vi "Init Control.vi"(5 "Group":refnum<class "Group DBL.lvclass">, 6 "Period ms":i64, 7 "VolatusAPI":refnum<class "VolatusAPI.lvclass">, 8 "error in (no error)":errorcluster, 9 "Control MsgQ":refnum<class "MessageQ.lvclass">, 10 "Config Element":refnum<class "Config Element.lvclass">, 11 "Valve in":refnum<class "BangBangControl.lvclass">) -> (0 "error out":errorcluster, 3 "Valve out":refnum<class "BangBangControl.lvclass">)   [LabVIEW 2020, in "VolatusControl.lvlib" / "BangBangControl.lvclass"]
uses:
  BangBangControl.lvclass
  lv-cdm/CDM-Config/Config Element/Config Element.lvclass
  Volatus/VolatusAPI/VolatusAPI.lvclass
  Volatus/MessageQ/MessageQ.lvclass
  lv-vecto/Vecto/Group DBL/Group DBL.lvclass
  C:/dev/lv20CE/relink/lv-vecto/Vecto/Group/Group.lvclass
  PV Calc.ctl
  BangBangControl.lvclass/BangBangControl.ctl
  VolatusControl.lvlib
  lv-vecto/Vecto/Group/Group.lvclass
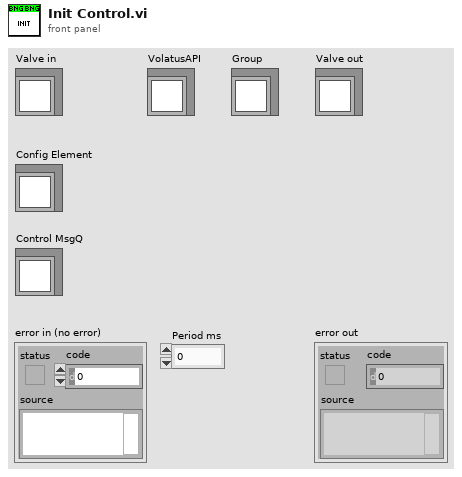
[diagram p1: front panel]
types:
  T1 = typedef "VolatusControl.lvlib/BangBangControl.lvclass/PV Calc.ctl" = enum16{"Average", "Median", "Max", "Min"}
  T2 = typedef "CDM-Config.lvlib/Value Type.ctl" = enum16{"String", "Number", "Bool", "Object", "Array"}
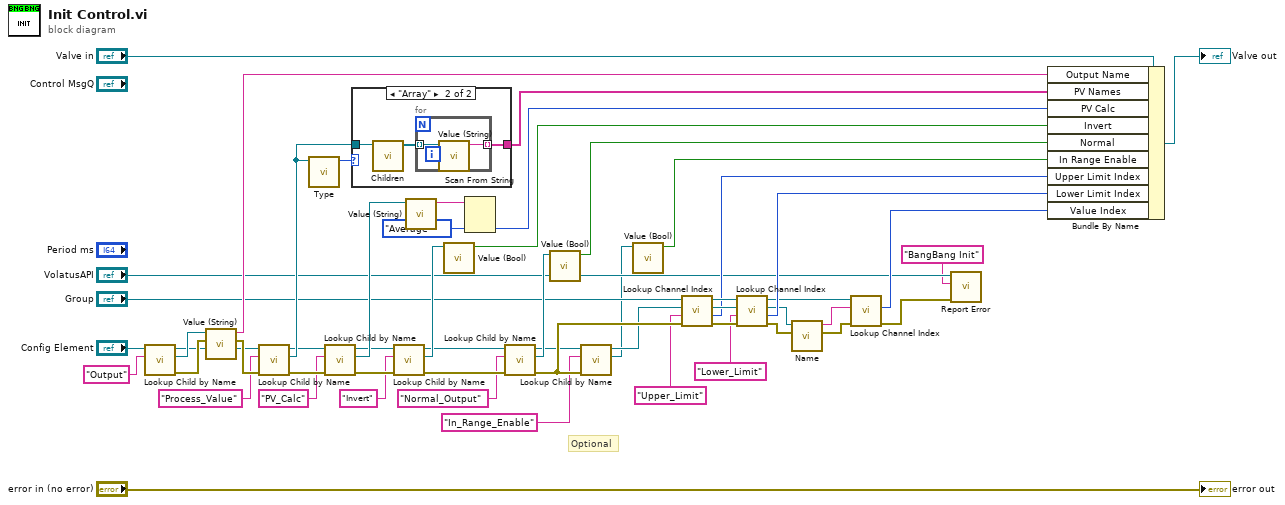
[diagram p0: block diagram]
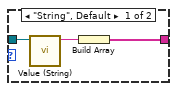
[diagram p2: hidden frame]
diagram:
  # "Optional"
  n1 = call "Lookup Child by Name.vi"("Name"="Output", "Config Element in"="Config Element") -> ("error out"=w44:errorcluster, "Child"=w45:refnum<class "Config Element.lvclass">, "Config Element out"=w41:refnum<class "Config Element.lvclass">)  [unwired: 6 in, 1 out]
  n2 = call "Value (String).vi"("error in (no error)"=w44, "Config Element in"=w45) -> ("error out"=w50:errorcluster, "String Value"=w42:string)  [unwired: 8 in]
  n3 = call "Lookup Child by Name.vi"("error in (no error)"=w50, "Name"="Process_Value", "Config Element in"=w41) -> ("error out"=w51:errorcluster, "Child"=w38:refnum<class "Config Element.lvclass">, "Config Element out"=w33:refnum<class "Config Element.lvclass">)  [unwired: 5 in, 1 out]
  n4 = call "Type.vi"("Config Element in"=w38) -> ("Value Type"=w39:T2)  [unwired: 9 in, 1 out]
  n5 = call "Lookup Child by Name.vi"("error in (no error)"=w51, "Name"="PV_Calc", "Config Element in"=w33) -> ("error out"=w52:errorcluster, "Child"=w32:refnum<class "Config Element.lvclass">, "Config Element out"=w29:refnum<class "Config Element.lvclass">)  [unwired: 5 in, 1 out]
  n6 = case shown="\"Array\"" w39 {
    tunnel: w38 -> [w57 w60]
    tunnel: [w55 w58] -> w37
    frame "String", Default {
      n7 = call "Value (String).vi"("Config Element in"=w57) -> ("String Value"=w56:string)  [unwired: 9 in, 1 out]
      n8 = Build Array(w56) -> (w55:string[])
    }
    frame "Array" {
      n9 = call "Children.vi"("Config Element in"=w60) -> ("Elements"=w59:refnum<class "Config Element.lvclass">[])  [unwired: 9 in, 1 out]
      n10 = for {
        tunnel: w59 -> [w62] mode=indexing
        tunnel: [w61] -> w58 mode=indexing
        n11 = call "Value (String).vi"("Config Element in"=w62) -> ("String Value"=w61:string)  [unwired: 9 in, 1 out]
      }
    }
  }
  n12 = call "Lookup Child by Name.vi"("error in (no error)"=w52, "Name"="Invert", "Config Element in"=w29) -> ("error out"=w53:errorcluster, "Child"=w28:refnum<class "Config Element.lvclass">, "Config Element out"=w24:refnum<class "Config Element.lvclass">)  [unwired: 5 in, 1 out]
  n13 = call "Value (String).vi"("Config Element in"=w32) -> ("String Value"=w36:string)  [unwired: 9 in, 1 out]
  n14 = call "Value (Bool).vi"("Config Element in"=w28) -> ("Bool Value"=w27:bool)  [unwired: 9 in, 1 out]
  n15 = Scan From String(input string=w36, default 1=PV_Calc."Average" ("PV Calc")) -> (output 1=w31:T1)  [unwired: 3 in, 3 out]
  n16 = call "Lookup Child by Name.vi"("error in (no error)"=w53, "Name"="Normal_Output", "Config Element in"=w24) -> ("error out"=w54:errorcluster, "Child"=w26:refnum<class "Config Element.lvclass">, "Config Element out"=w5:refnum<class "Config Element.lvclass">)  [unwired: 5 in, 1 out]
  n17 = call "Value (Bool).vi"("Config Element in"=w26) -> ("Bool Value"=w23:bool)  [unwired: 9 in, 1 out]
  n18 = call "Lookup Child by Name.vi"("error in (no error)"=w54, "Name"="In_Range_Enable", "Config Element in"=w5) -> ("Child"=w2:refnum<class "Config Element.lvclass">, "Config Element out"=w3:refnum<class "Config Element.lvclass">)  [unwired: 5 in, 2 out]
  n19 = call "Value (Bool).vi"("Config Element in"=w2) -> ("Bool Value"=w1:bool)  [unwired: 9 in, 1 out]
  n20 = call "Lookup Channel Index.vi"("error in (no error)"=w54, "Meta Value"="Upper_Limit", "Config Element in"=w3, "Group in"="Group") -> ("error out"=w19:errorcluster, "Index"=w17:i32, "Config Element"=w18:refnum<class "Config Element.lvclass">, "Group"=w20:refnum<class "Group DBL.lvclass">)  [unwired: 4 in]
  n21 = call "Lookup Channel Index.vi"("error in (no error)"=w19, "Meta Value"="Lower_Limit", "Config Element in"=w18, "Group in"=w20) -> ("error out"=w10:errorcluster, "Index"=w15:i32, "Config Element"=w12:refnum<class "Config Element.lvclass">, "Group"=w11:refnum<class "Group DBL.lvclass">)  [unwired: 4 in]
  n22 = call "Name.vi"("error in (no error)"=w10, "Config Element in"=w12) -> ("error out"=w13:errorcluster, "Name"=w14:string)  [unwired: 8 in]
  n23 = call "Lookup Channel Index.vi"("error in (no error)"=w13, "Channel Name"=w14, "GroupAbstract in"=w11) -> ("error out"=w7:errorcluster, "Index"=w9:i32)  [unwired: 6 in, 1 out]
  n24 = call "Report Error.vi"("error in (no error)"=w7, "Context"="BangBang Init", "VolatusAPI in"="VolatusAPI") -> ()  [unwired: 7 in, 2 out]
  n25 = Bundle By Name(cluster="Valve in", "Output Name"=w42, "PV Names"=w37, "PV Calc"=w31, "Invert"=w27, "Normal"=w23, "In Range Enable"=w1, "Upper Limit Index"=w17, "Lower Limit Index"=w15, "Value Index"=w9) -> (→"Valve out":refnum<class "BangBangControl.lvclass">)
  "error out" <- "error in (no error)"
